vi "subVI2.vi"(6 "Duty Cycle (0-1)":dbl, 8 "Serial Port":refnum<visa-resource-name>="COM4", 9 "stop":bool, 10 "B":bool, 11 "A":bool) -> (1 "x/y":dbl(knob) scale=0.0..200.0, 2 "Pulse Time (us)":u16, 3 "Pulse Count":i32)   [LabVIEW 2020]
uses:
  <vilib>/MakerHub/LINX/Public/Peripherals/Digital/Digital Write N Chans.vi
  <vilib>/MakerHub/LINX/Public/Utilities/Open Serial.vi
  <vilib>/MakerHub/LINX/Public/Peripherals/PWM/PWM Set Duty Cycle 1 Chan.vi
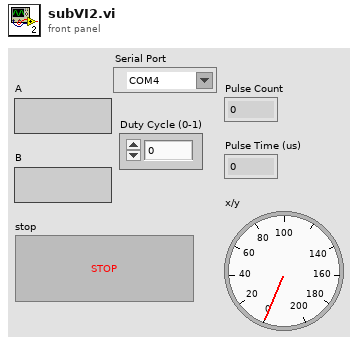
[diagram p1: front panel]
types:
  T1 = enum8{"Channel 0 (pins A8 & A9)", "Channel 1 (pins A10 & A11)", "Channel 2 (pins 2 & 3)", "Channel 3 (pins 18 & 19)", "Channel 4 (pins 20 & 21)"}
  T2 = typedef "LMH-LINX.lvlib/LINX Ref.ctl" = cluster{"IO":T3, "Interface":T4, "LINX Device Config":T5}
  T3 = typedef "LMH-LINX.lvlib/Platform.ctl" = enum16{"Remote", "Local"}
  T4 = typedef "LMH-LINX.lvlib/Interface.ctl" = enum16{"Serial", "TCP"}
  T5 = typedef "LMH-LINX.lvlib/Device.lvlib/LINX Device Config.ctl" = cluster{"Interface":T4, "COM Port":refnum<visa-resource-name>, "TCP Configuration":T6, "Device Family":u8, "Device ID":u8, "Device Name":string, "TCP Ref":refnum<k5>, "Channels":T7}
  T6 = typedef "LMH-LINX.lvlib/Device.lvlib/TCP Config.ctl" = cluster{"IP Address":string, "Port":u16}
  T7 = typedef "LMH-LINX.lvlib/Channels.ctl" = cluster{"DI":u8[], "DO":u8[], "AI":u8[], "AO":u8[], "PWM":u8[], "QE":u8[], "UART":u8[], "I2C 2":u8[], "SPI":u8[], "CAN":u8[], "Servo":u8[], "AI Ref (V)":dbl, "AI Resolution (Bits)":u8, "AO Ref (V)":dbl, "AO Resolution (Bits)":u8}
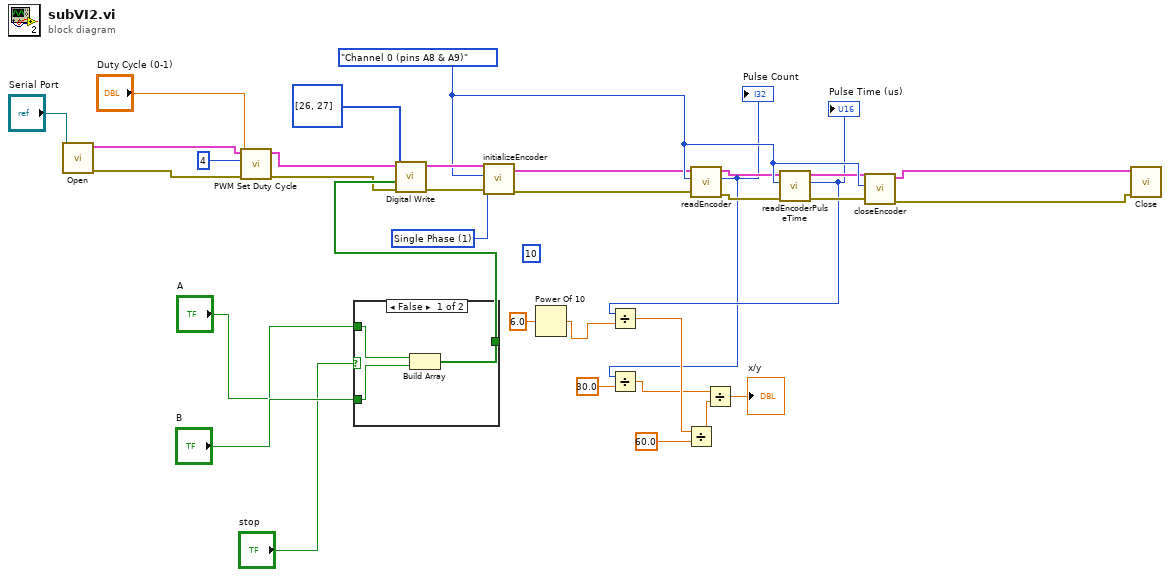
[diagram p0: block diagram]
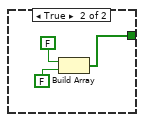
[diagram p2: hidden frame]
diagram:
  (unwired) 10
  w19 = u8 1 items=["Single Phase"=1, "Single Phase Double Resolution"=2, "Quadrature"=3] ("Encoder Type")
  w26 = T1."Channel 0 (pins A8 & A9)" ("Channel")
  n1 = call-poly <vilib>:"Open.vi"("Serial Port"="Serial Port") -> ("Error Out"=w5:errorcluster, "LINX Resource"=w6:T2)  [unwired: 8 in, 1 out]
  n2 = call-poly <vilib>:"PWM Set Duty Cycle.vi"("Error In"=w5, "Duty Cycle (0-1)"="Duty Cycle (0-1)", "PWM Channel"=u8 4, "LINX Resource"=w6) -> ("Error Out"=w3:errorcluster, "LINX Resource"=w4:T2)  [unwired: 6 in]
  n3 = case shown="False" "stop" {
    tunnel: "A" -> [w37 _]
    tunnel: "B" -> [w36 _]
    tunnel: [w35 w38] -> w9
    frame False {
      n4 = Build Array(w37, w36) -> (w35:bool[])
    }
    frame True {
      n5 = Build Array(FALSE, FALSE) -> (w38:bool[])
    }
  }
  n6 = call-poly <vilib>:"Digital Write.vi"("Error In"=w3, "Values"=w9, "DO Channels"=u8[] [26, 27], "LINX Resource"=w4) -> ("Error Out"=w27:errorcluster, "LINX Resource"=w28:T2)  [unwired: 6 in]
  n7 = call <vilib>:"initializeEncoder.vi"("Error In"=w27, "Encoder Type"=w19, "Channel"=w26, "LINX Resource In"=w28) -> ("Error Out"=w23:errorcluster, "LINX Resource Out"=w24:T2)  [unwired: 6 in]
  n8 = Power Of 10(x=6.0) -> (10^x=w7:dbl)
  n9 = call <vilib>:"readEncoder.vi"("Error In"=w23, "Channel"=w26, "LINX Resource In"=w24) -> ("Error Out"=w22:errorcluster, "Pulse Count"=w14:i32, "LINX Resource Out"=w25:T2)  [unwired: 6 in]
  "Pulse Count" <- w14
  n10 = Divide(x=w14, y=30.0) -> (x/y=w13:dbl)
  n11 = call <vilib>:"readEncoderPulseTime.vi"("Error In"=w22, "Channel"=w26, "LINX Resource In"=w25) -> ("Error Out"=w21:errorcluster, "Pulse Time (us)"=w16:u16, "LINX Resource Out"=w20:T2)  [unwired: 6 in]
  "Pulse Time (us)" <- w16
  n12 = Divide(x=w16, y=w7) -> (x/y=w15:dbl)
  n13 = Divide(x=w15, y=60.0) -> (x/y=w12:dbl)
  n14 = Divide(x=w13, y=w12) -> (x/y=→"x/y":dbl)
  n15 = call <vilib>:"closeEncoder.vi"("Error In"=w21, "Channel"=w26, "LINX Resource In"=w20) -> ("Error Out"=w32:errorcluster, "LINX Resource Out"=w31:T2)  [unwired: 7 in]
  n16 = call <vilib>:"Close.vi"("Error In"=w32, "LINX Resource"=w31) -> ()  [unwired: 9 in, 1 out]
